vi "Auto - Drive a Distance (SubVI).vi"(5 "Override Drive Gain":bool, 7 "Drive PID":T2={"Auton Prop Drive Gain"=0.005, "Auton Int Drive Gain"=0.02, "Auton Deriv Drive Gain"=0.0, "I Output Limit"=0.15}, 8 "Constant cluster In":T3 {"15. Center-Center Sector Distance" format="%_6f"; "14. Inches / Tick Drivetrain" format="%_6f"; "13. Auton I Output Limit Drive Straight Gain" format="%_6f"; "12. Auton Deriv Drive Straight Gain" format="%_6f"; "11. Auton Int Drive Straight Gain" format="%_6f"; "10. Auton Prop Drive Straight Gain" format="%_6f"; "9. Auton I Output Limit Turn Gain" format="%_6f"; "8. Auton Deriv Turn Gain" format="%_6f"; "7. Auton Int Turn Gain" format="%_6f"; "1. Auton Prop Drive Gain" format="%_6f"; "2. Auton Int Drive Gain" format="%_6f"; "3. Auton Deriv Drive Gain" format="%_6f"; "4. I Output Drive  Limit" format="%_6f"; "5. Auto Drive Cheat (%)" format="%_6f"; "6. Auton Prop Turn Gain" format="%_6f"}, 9 "Auton Input Cluster In":T4, 10 "Sensors In":T1) -> (0 "Constant cluster Out":T3 {"15. Center-Center Sector Distance" format="%_6f"; "14. Inches / Tick Drivetrain" format="%_6f"; "13. Auton I Output Limit Drive Straight Gain" format="%_6f"; "12. Auton Deriv Drive Straight Gain" format="%_6f"; "11. Auton Int Drive Straight Gain" format="%_6f"; "10. Auton Prop Drive Straight Gain" format="%_6f"; "9. Auton I Output Limit Turn Gain" format="%_6f"; "8. Auton Deriv Turn Gain" format="%_6f"; "7. Auton Int Turn Gain" format="%_6f"; "1. Auton Prop Drive Gain" format="%_6f"; "2. Auton Int Drive Gain" format="%_6f"; "3. Auton Deriv Drive Gain" format="%_6f"; "4. I Output Drive  Limit" format="%_6f"; "5. Auto Drive Cheat (%)" format="%_6f"; "6. Auton Prop Turn Gain" format="%_6f"}, 1 "Auton Input Cluster Out":T4, 2 "Sensors Out":T1, 3 "Drive Output (%)":dbl)   [LabVIEW 2020]
uses:
  TypeDefs/Auton Cluster Typedef.ctl
  Disabled/Constant VI_s/Disabled - Constant Cluster Typedef.ctl
  TypeDefs/Sensor TypeDef.ctl
panel:
  out "Waveform Chart":dbl(graph)
  # "Tune Drive Gains"
  # "Outputs"
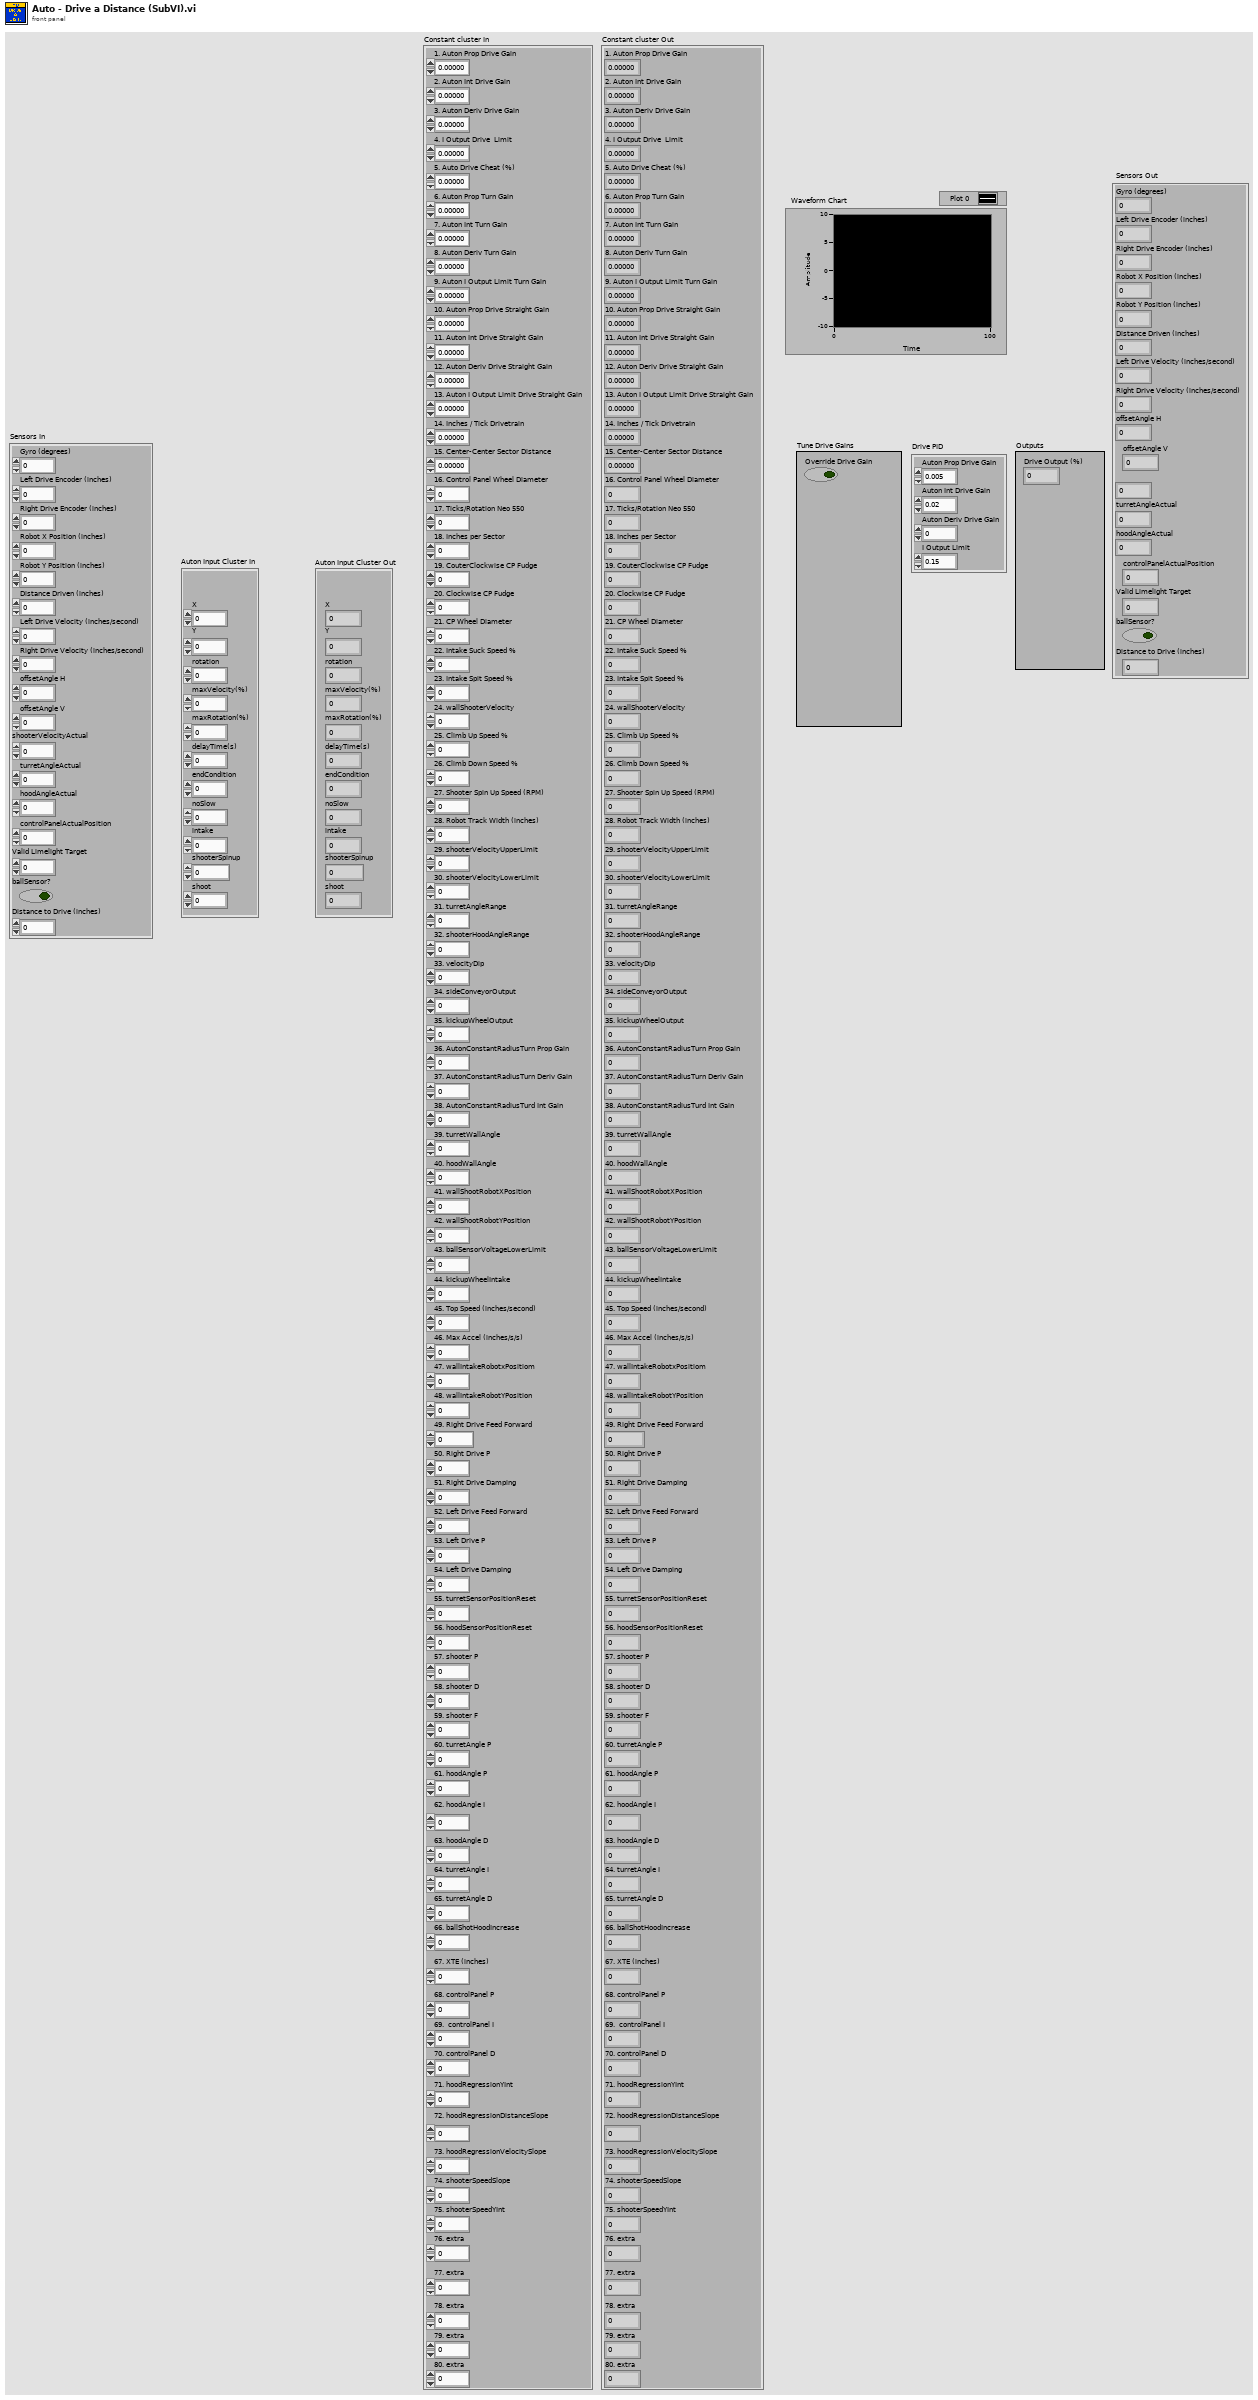
[diagram p1: front panel]
types:
  T1 = typedef "Sensor TypeDef.ctl" = cluster{"Gyro (degrees)":dbl, "Left Drive Encoder (inches)":dbl, "Right Drive Encoder (inches)":dbl, "Robot X Position (inches)":dbl, "Robot Y Position (inches)":dbl, "Distance Driven (inches)":dbl, "Left Drive Velocity (inches/second)":dbl, "Right Drive Velocity (inches/second)":dbl, "offsetAngle H":dbl, "offsetAngle V":dbl, "shooterVelocityActual":dbl, "turretAngleActual":dbl, "hoodAngleActual":dbl, "controlPanelActualPosition":dbl, "Valid Limelight Target":dbl, "ballSensor?":bool, "Distance to Drive (inches)":dbl}
  T2 = cluster{"Auton Prop Drive Gain":dbl, "Auton Int Drive Gain":dbl, "Auton Deriv Drive Gain":dbl, "I Output Limit":dbl}
  T3 = typedef "Disabled - Constant Cluster Typedef.ctl" = cluster{"1. Auton Prop Drive Gain":dbl, "2. Auton Int Drive Gain":dbl, "3. Auton Deriv Drive Gain":dbl, "4. I Output Drive  Limit":dbl, "5. Auto Drive Cheat (%)":dbl, "6. Auton Prop Turn Gain":dbl, "7. Auton Int Turn Gain":dbl, "8. Auton Deriv Turn Gain":dbl, "9. Auton I Output Limit Turn Gain":dbl, "10. Auton Prop Drive Straight Gain":dbl, "11. Auton Int Drive Straight Gain":dbl, "12. Auton Deriv Drive Straight Gain":dbl, "13. Auton I Output Limit Drive Straight Gain":dbl, "14. Inches / Tick Drivetrain":dbl, "15. Center-Center Sector Distance":dbl, "16. Control Panel Wheel Diameter":dbl, "17. Ticks/Rotation Neo 550":dbl, "18. Inches per Sector":dbl, "19. CouterClockwise CP Fudge":dbl, "20. Clockwise CP Fudge":dbl, "21. CP Wheel Diameter":dbl, "22. Intake Suck Speed %":dbl, "23. Intake Spit Speed %":dbl, "24. wallShooterVelocity":dbl, "25. Climb Up Speed %":dbl, "26. Climb Down Speed %":dbl, "27. Shooter Spin Up Speed (RPM)":dbl, "28. Robot Track Width (inches)":dbl, "29. shooterVelocityUpperLimit":dbl, "30. shooterVelocityLowerLimit":dbl, "31. turretAngleRange":dbl, "32. shooterHoodAngleRange":dbl, "33. velocityDip":dbl, "34. sideConveyorOutput":dbl, "35. kickupWheelOutput":dbl, "36. AutonConstantRadiusTurn Prop Gain":dbl, "37. AutonConstantRadiusTurn Deriv Gain":dbl, "38. AutonConstantRadiusTurd Int Gain":dbl, "39. turretWallAngle":dbl, "40. hoodWallAngle":dbl, "41. wallShootRobotXPosition":dbl, "42. wallShootRobotYPosition":dbl, "43. ballSensorVoltageLowerLimit":dbl, "44. kickupWheelIntake":dbl, "45. Top Speed (inches/second)":dbl, "46. Max Accel (inches/s/s)":dbl, "47. wallIntakeRobotxPositiom":dbl, "48. wallIntakeRobotYPosition":dbl, "49. Right Drive Feed Forward":dbl, "50. Right Drive P":dbl, "51. Right Drive Damping":dbl, "52. Left Drive Feed Forward":dbl, "53. Left Drive P":dbl, "54. Left Drive Damping":dbl, "55. turretSensorPositionReset":dbl, "56. hoodSensorPositionReset":dbl, "57. shooter P":dbl, "58. shooter D":dbl, "59. shooter F":dbl, "60. turretAngle P":dbl, "61. hoodAngle P":dbl, "62. hoodAngle I":dbl, "63. hoodAngle D":dbl, "64. turretAngle I":dbl, "65. turretAngle D":dbl, "66. ballShotHoodIncrease":dbl, "67. XTE (inches)":dbl, "68. controlPanel P":dbl, "69.  controlPanel I":dbl, "70. controlPanel D":dbl, "71. hoodRegressionYInt":dbl, "72. hoodRegressionDistanceSlope":dbl, "73. hoodRegressionVelocitySlope":dbl, "74. shooterSpeedSlope":dbl, "75. shooterSpeedYInt":dbl, "76. extra":dbl, "77. extra":dbl, "78. extra":dbl, "79. extra":dbl, "80. extra":dbl}
  T4 = typedef "Auton Cluster Typedef.ctl" = cluster{"rotation":dbl, "maxVelocity(%)":dbl, "delayTime(s)":dbl, "endCondition":dbl, "noSlow":dbl, "intake":dbl, "shooterSpinup":dbl, "shoot":dbl, "X":dbl, "Y":dbl, "maxRotation(%)":dbl}
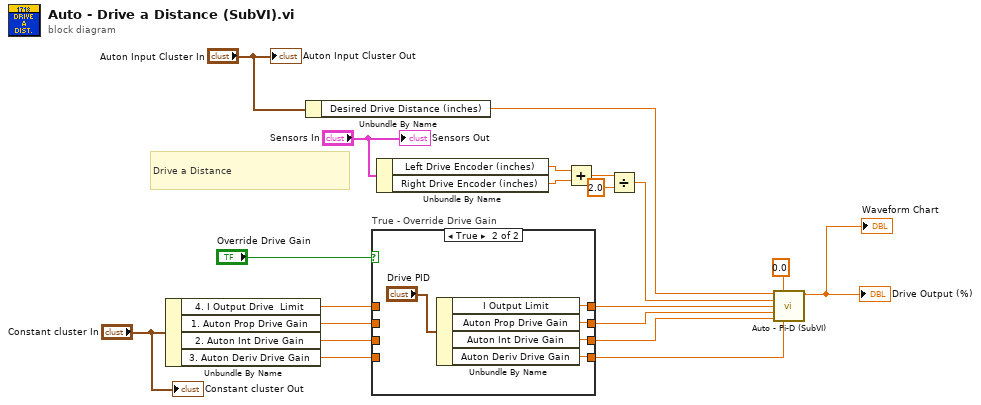
[diagram p0: block diagram]
diagram:
  # "Drive a Distance"
  n1 = Unbundle By Name("Constant cluster In") -> ("4. I Output Drive  Limit"=w10:dbl, "1. Auton Prop Drive Gain"=w11:dbl, "2. Auton Int Drive Gain"=w12:dbl, "3. Auton Deriv Drive Gain"=w15:dbl)
  n2 = Unbundle By Name("Auton Input Cluster In") -> ("Desired Drive Distance (inches)"=w3:dbl)
  n3 = case "True - Override Drive Gain" shown="True" "Override Drive Gain" {
    tunnel: w10 -> [w24 _]
    tunnel: w11 -> [w23 _]
    tunnel: w12 -> [w22 _]
    tunnel: [w24 w28] -> w16
    tunnel: [w23 w27] -> w17
    tunnel: [w22 w26] -> w18
    tunnel: [w21 w25] -> w19
    tunnel: w15 -> [w21 _]
    frame False {
    }
    frame True {
      n4 = Unbundle By Name("Drive PID") -> ("I Output Limit"=w28:dbl, "Auton Prop Drive Gain"=w27:dbl, "Auton Int Drive Gain"=w26:dbl, "Auton Deriv Drive Gain"=w25:dbl)
    }
  }
  n5 = Unbundle By Name("Sensors In") -> ("Left Drive Encoder (inches)"=w7:dbl, "Right Drive Encoder (inches)"=w6:dbl)
  n6 = Add(x=w7, y=w6) -> (x+y=w5:dbl)
  n7 = Divide(x=w5, y=2.0) -> (x/y=w2:dbl)
  n8 = call "Auto - Pi-D (SubVI).vi"("Desired Value"=w3, "I Windup Limit"=0.0, "Actual Value"=w2, "I Output Limit"=w16, "Prop Gain"=w17, "Int Gain"=w18, "Deriv Gain"=w19) -> ("Output"=→"Drive Output (%)" →"Waveform Chart":dbl)  [unwired: 8 in]
  "Auton Input Cluster Out" <- "Auton Input Cluster In"
  "Constant cluster Out" <- "Constant cluster In"
  "Sensors Out" <- "Sensors In"
